vi "CRYHeader x-y settings full.vi"(9 "x-y settings array":T1=[{"x col"=0, "x data type"=0, "x axis type"=0, "x prefix"="", "x unit"="", "x db ref"=0.0, "y col"=0, "Name:"="", "phase incl"=FALSE, "ym data type"=0, "ym axis type"=0, "ym prefix"="", "ym unit"="", "ym db ref"=0.0, "yp data type"=0, "yp axis type"=0, "yp prefix"="", "yp unit"="", "yp db ref"=0.0}] {"yp db ref" format="%.2f"; "ym db ref" format="%.2f"; "x db ref" format="%.2f"}, 10 "Main info cluster":T2, 11 "Row length":i32) -> (0 "dB ref row out":string[](array[string]), 1 "Axis type row out":string[](array[string]), 2 "Data type row out":string[](array[string]), 3 "Name row out":string[](array[string]))   [LabVIEW 2013]
uses:
  Control/CRYImp wiz main info.ctl
  Control/CRYx-y settings array.ctl
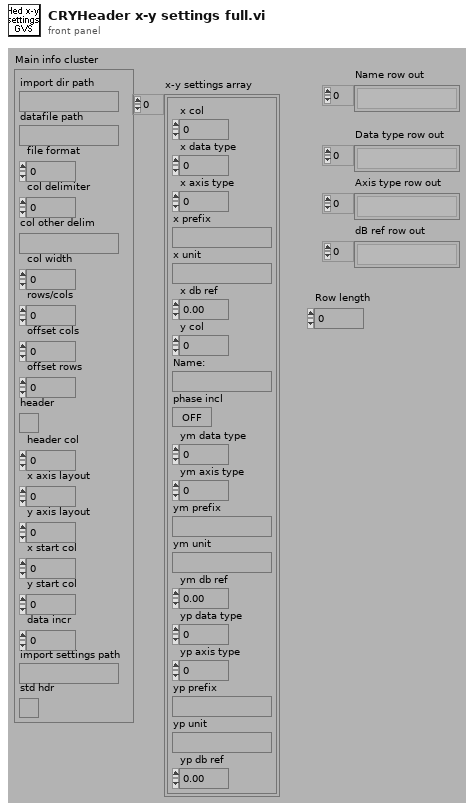
[diagram p1: front panel]
types:
  T1 = typedef "CRYx-y settings array.ctl" = cluster{"x col":i32, "x data type":u16, "x axis type":u16, "x prefix":string, "x unit":string, "x db ref":dbl, "y col":i32, "Name:":string, "phase incl":bool, "ym data type":u16, "ym axis type":u16, "ym prefix":string, "ym unit":string, "ym db ref":dbl, "yp data type":u16, "yp axis type":u16, "yp prefix":string, "yp unit":string, "yp db ref":dbl}[]
  T2 = typedef "CRYImp wiz main info.ctl" = cluster{"import dir path":path, "datafile path":path, "file format":i32, "col delimiter":i32, "col other delim":string, "col width":i32, "rows/cols":i32, "offset cols":i32, "offset rows":i32, "header":bool, "header col":i32, "x axis layout":i32, "y axis layout":i32, "x start col":i32, "y start col":i32, "data incr":i32, "import settings path":path, "std hdr":bool}
  T3 = cluster{"x col":i32, "x data type":u16, "x axis type":u16, "x prefix":string, "x unit":string, "x db ref":dbl, "y col":i32, "Name:":string, "phase incl":bool, "ym data type":u16, "ym axis type":u16, "ym prefix":string, "ym unit":string, "ym db ref":dbl, "yp data type":u16, "yp axis type":u16, "yp prefix":string, "yp unit":string, "yp db ref":dbl}[]
  T4 = cluster{"x Data type":string, "x Axis type":string, "x dB ref":string, "y Data type":string, "y Axis type":string, "y dB ref":string, "z Data type":string, "z Axis type":string, "z dB ref":string}
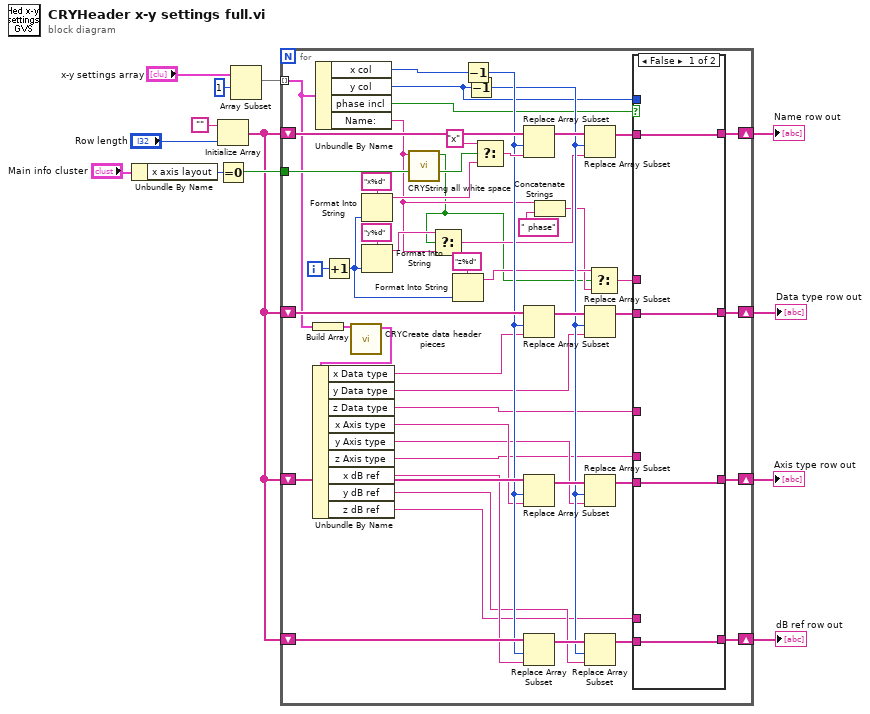
[diagram p0: block diagram]
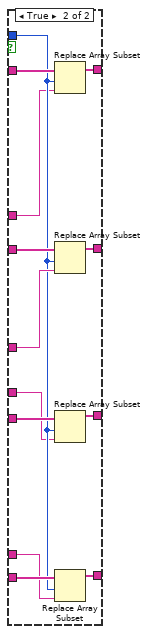
[diagram p2: hidden frame]
diagram:
  n1 = Unbundle By Name("Main info cluster") -> ("x axis layout"=w5:i32)
  n2 = Initialize Array("", "Row length") -> (w3:string[])
  n3 = Equal To 0?(x=w5) -> (x = 0?=w6:bool)
  n4 = Array Subset(array="x-y settings array", index=1 ("Array Index")) -> (w11:T1)  [unwired: 1 in]
  n5 = for {
    tunnel: w11 -> [w35] mode=indexing
    shift-right: [w43] -> w13
    shift-left: w3 -> [w63]
    tunnel: w6 -> [w57]
    shift-right: [w41] -> w4
    shift-left: w3 -> [w53]
    shift-right: [w39] -> w2
    shift-left: w3 -> [w49]
    shift-right: [w37] -> w1
    shift-left: w3 -> [w48]
    i -> [w60]
    n6 = Build Array(w35) -> (w34:T3)
    n7 = Unbundle By Name(w35) -> ("x col"=w58:i32, "y col"=w45:i32, "phase incl"=w36:bool, "Name:"=w15:string)
    n8 = Increment(x=w60) -> (x+1=w23:i32)
    n9 = call "CRYCreate data header pieces.vi"("x-y settings array"=w34) -> ("Descriptive strings"=w33:T4)  [unwired: 10 in]
    n10 = Unbundle By Name(w33) -> ("x Data type"=w32:string, "y Data type"=w31:string, "z Data type"=w30:string, "x Axis type"=w29:string, "y Axis type"=w28:string, "z Axis type"=w27:string, "x dB ref"=w26:string, "y dB ref"=w25:string, "z dB ref"=w24:string)
    n11 = Format Into String(format string="x%d", w23) -> (resulting string=w56:string)  [unwired: 2 in, 1 out]
    n12 = Format Into String(format string="y%d", w23) -> (resulting string=w21:string)  [unwired: 2 in, 1 out]
    n13 = call "CRYString all white space.vi"("String"=w15) -> ("Nothing but white space?"=w14:bool)  [unwired: 10 in]
    n14 = Select(t=w21, s=w14, f=w15) -> (s? t:f=w18:string)
    n15 = Format Into String(format string="z%d", w23) -> (resulting string=w20:string)  [unwired: 2 in, 1 out]
    n16 = Decrement(x=w58) -> (x-1=w47:i32)
    n17 = Decrement(x=w45) -> (x-1=w46:i32)
    n18 = Select(t="x", s=w57, f=w56) -> (s? t:f=w54:string)
    n19 = Replace Array Subset(array=w63, new element=w54, index=w47) -> (w59:string[])
    n20 = Replace Array Subset(array=w53, new element=w32, index=w47) -> (w52:string[])
    n21 = Replace Array Subset(array=w49, new element=w29, index=w47) -> (w51:string[])
    n22 = Replace Array Subset(array=w48, new element=w26, index=w47) -> (w50:string[])
    n23 = Concatenate Strings(w15, " phase") -> (w17:string)
    n24 = Replace Array Subset(array=w59, new element=w18, index=w46) -> (w44:string[])
    n25 = Replace Array Subset(array=w52, new element=w31, index=w46) -> (w42:string[])
    n26 = Replace Array Subset(array=w51, new element=w28, index=w46) -> (w40:string[])
    n27 = Replace Array Subset(array=w50, new element=w25, index=w46) -> (w38:string[])
    n28 = Select(t=w20, s=w14, f=w17) -> (s? t:f=w16:string)
    n29 = case shown="False" w36 {
      tunnel: w45 -> [_ w71]
      tunnel: w44 -> [w67 w80]
      tunnel: [w67 w79] -> w43
      tunnel: w42 -> [w66 w78]
      tunnel: [w66 w77] -> w41
      tunnel: w40 -> [w65 w76]
      tunnel: [w65 w75] -> w39
      tunnel: w38 -> [w64 w74]
      tunnel: [w64 w73] -> w37
      tunnel: w30 -> [_ w72]
      tunnel: w27 -> [_ w70]
      tunnel: w24 -> [_ w69]
      tunnel: w16 -> [_ w68]
      frame False {
      }
      frame True {
        n30 = Replace Array Subset(array=w80, new element=w68, index=w71) -> (w79:string[])
        n31 = Replace Array Subset(array=w78, new element=w72, index=w71) -> (w77:string[])
        n32 = Replace Array Subset(array=w76, new element=w70, index=w71) -> (w75:string[])
        n33 = Replace Array Subset(array=w74, new element=w69, index=w71) -> (w73:string[])
      }
    }
  }
  "Name row out" <- w13
  "Axis type row out" <- w2
  "dB ref row out" <- w1
  "Data type row out" <- w4
